vi "Compare Bitpacked Channels.vi"(7 "expected values":string[][](array[string]), 8 "error in (no error)":errorcluster, 10 "bitfile scalars in":T1[](array[typedef]), 11 "FPGA addon refnum in":T3 format="%.0x") -> (0 "error out":errorcluster, 2 "equal":bool)   [LabVIEW 2018, in "FPGA Addon Bitfile Reload Unit Tests.lvclass"]
uses:
  FPGA Addon Bitfile Reload Unit Tests.lvclass
  <vilib>/NI Veristand/Custom Device API/Custom Device Item Ref.ctl
  APIs/Scripting API/TypeDefs/Output Scalar Data.ctl
  Addon/Addon Shared/Types/Data Type.ctl
  Addon/Addon Shared/SubVIs/Constants.vi
  <vilib>/NI/NI VeriStand Advanced SysDef API/_SubVIs/SysDef.Search.Name.vi
  <vilib>/NI/NI VeriStand Advanced SysDef API/_SubVIs/SysDef.Search.GUIDs.vi
  <vilib>/NI/NI VeriStand Advanced SysDef API/SysDef API/Advanced System Definition.lvlib
  Addon/Addon Shared/FPGA Addon Shared.lvlib
  <vilib>/NI Veristand/Custom Device API/Custom Device API.lvlib
  APIs/Scripting API/Scripting API.lvlib
panel:
  out "Array":string[](array[string])
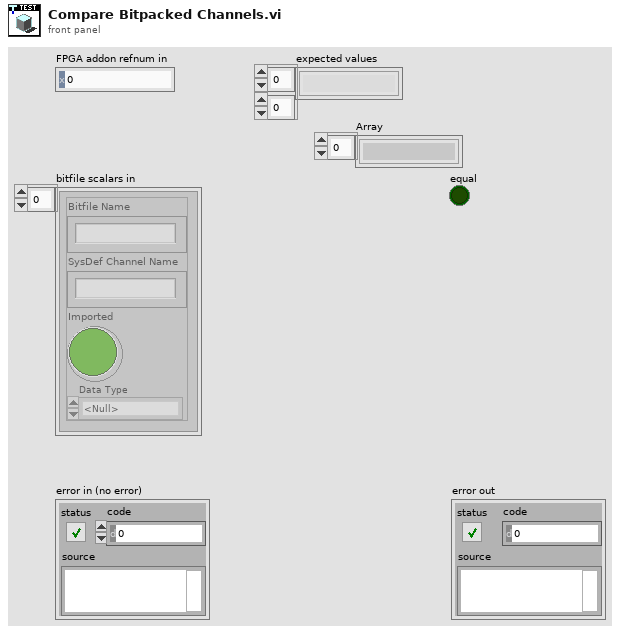
[diagram p1: front panel]
types:
  T1 = typedef "Scripting API.lvlib/Output Scalar Data.ctl" = cluster{"Bitfile Name":string, "SysDef Channel Name":string, "Imported":bool, "Data Type":T2}
  T2 = typedef "FPGA Addon Shared.lvlib/Data Type.ctl" = enum8{"<Null>", "I8", "I16", "I32", "I64", "U8", "U16", "U32", "U64", "SGL", "Boolean", "Analog PWM In Settings", "Analog PWM In", "Digital PWM In Settings", "Digital PWM In", "Digital PWM Out", "Sine Out", "FXP+/-24.5", "FXP+/-16.5", "FXP+/-32.8", "FXP+/-64.32", "FXP+/-16.7", "FXP+/-20.5", "FXP+/-27.5", "FXP+/-32.16", "FXP+16.3", "FXP+18.3", "Digital Static In", "Digital Static Out", "Digital Static In Settings", "Digital WSS Out", "Quad Encoder Settings", "Quad Encoder In", "Group"}
  T3 = typedef "Custom Device API.lvlib/Custom Device Item Ref.ctl" = u64
  T4 = typedef "Custom Device API.lvlib/Custom Device Item Info.ctl" = cluster{"Name":string, "Is Channel":bool, "GUID":string, "Is Waveform":bool}
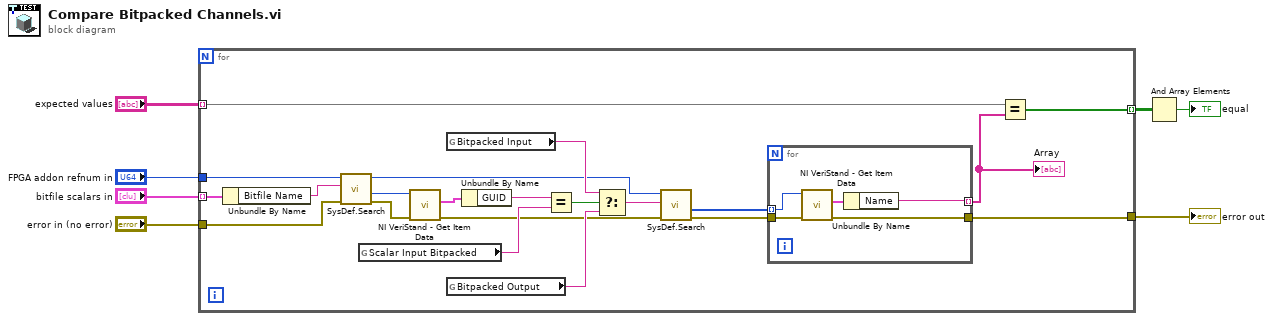
[diagram p0: block diagram]
diagram:
  n1 = for {
    tunnel: "error in (no error)" -> [w28]
    tunnel: "bitfile scalars in" -> [w27] mode=indexing
    tunnel: "FPGA addon refnum in" -> [w25]
    tunnel: [w11] -> w4
    tunnel: "expected values" -> [w10] mode=indexing
    tunnel: [w8] -> w2 mode=indexing
    n2 = Unbundle By Name(w27) -> ("Bitfile Name"=w26:string)
    n3 = call-poly <vilib>:"SysDef.Search.vi"("error in (no error)"=w28, "Name"=w26, "nodeID"=w25) -> ("error out"=w23:errorcluster, "Value out"=w24:u64, "nodeID out"=w15:u64)  [unwired: 5 in, 1 out]
    n4 = global read "Constants.vi" "Scalar Input Bitpacked"() -> (w20:string)
    n5 = call <vilib>:"NI VeriStand - Get Item Data.vi"("error in (no error)"=w23, "Item Ref in"=w24) -> ("error out"=w14:errorcluster, "Item Info"=w22:T4)  [unwired: 6 in, 2 out]
    n6 = global read "Constants.vi" "Bitpacked Input"() -> (w18:string)
    n7 = global read "Constants.vi" "Bitpacked Output"() -> (w17:string)
    n8 = Unbundle By Name(w22) -> ("GUID"=w21:string)
    n9 = Equal?(x=w21, y=w20) -> (x = y?=w19:bool)
    n10 = Select(t=w18, s=w19, f=w17) -> (s? t:f=w16:string)
    n11 = call-poly <vilib>:"SysDef.Search.vi"("error in (no error)"=w14, "GUID"=w16, "nodeID"=w15) -> ("error out"=w12:errorcluster, "Values Out"=w13:u64[])  [unwired: 5 in, 2 out]
    n12 = for {
      tunnel: w13 -> [w32] mode=indexing
      tunnel: w12 -> [w33]
      tunnel: [w30] -> w9 mode=indexing
      tunnel: [w29] -> w11
      n13 = call <vilib>:"NI VeriStand - Get Item Data.vi"("error in (no error)"=w33, "Item Ref in"=w32) -> ("error out"=w29:errorcluster, "Item Info"=w31:T4)  [unwired: 6 in, 2 out]
      n14 = Unbundle By Name(w31) -> ("Name"=w30:string)
    }
    "Array" <- w9
    n15 = Equal?(x=w10, y=w9) -> (x = y?=w8:bool[])
  }
  "error out" <- w4
  n16 = And Array Elements(Boolean array=w2) -> (logical AND=→"equal":bool)
